vi "majchambre.vi"() -> ()   [LabVIEW 2015]
uses:
  <vilib>/httpClient/LabVIEWHTTPClient.lvlib
panel:
  in  "OK Button 4":bool
  in  "OK Button 3":bool
  in  "String 2":string
  in  "String":string
  in  "Combo Box":string(combo)
  in  "OK Button 2":bool
  in  "OK Button":bool
  # "Choisir  chambre"
  # "Nom chambre"
  # "Description chambre"
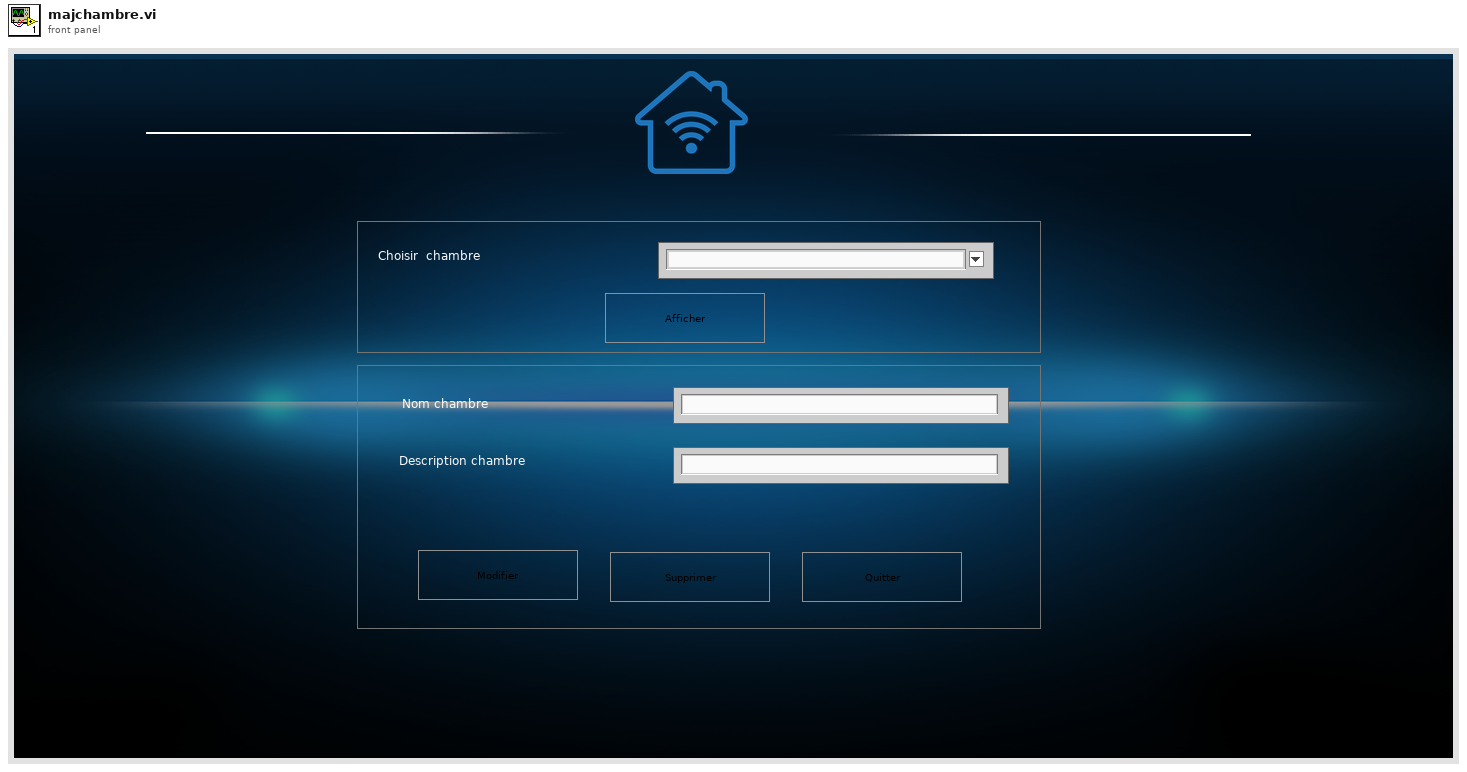
[diagram p1: front panel]
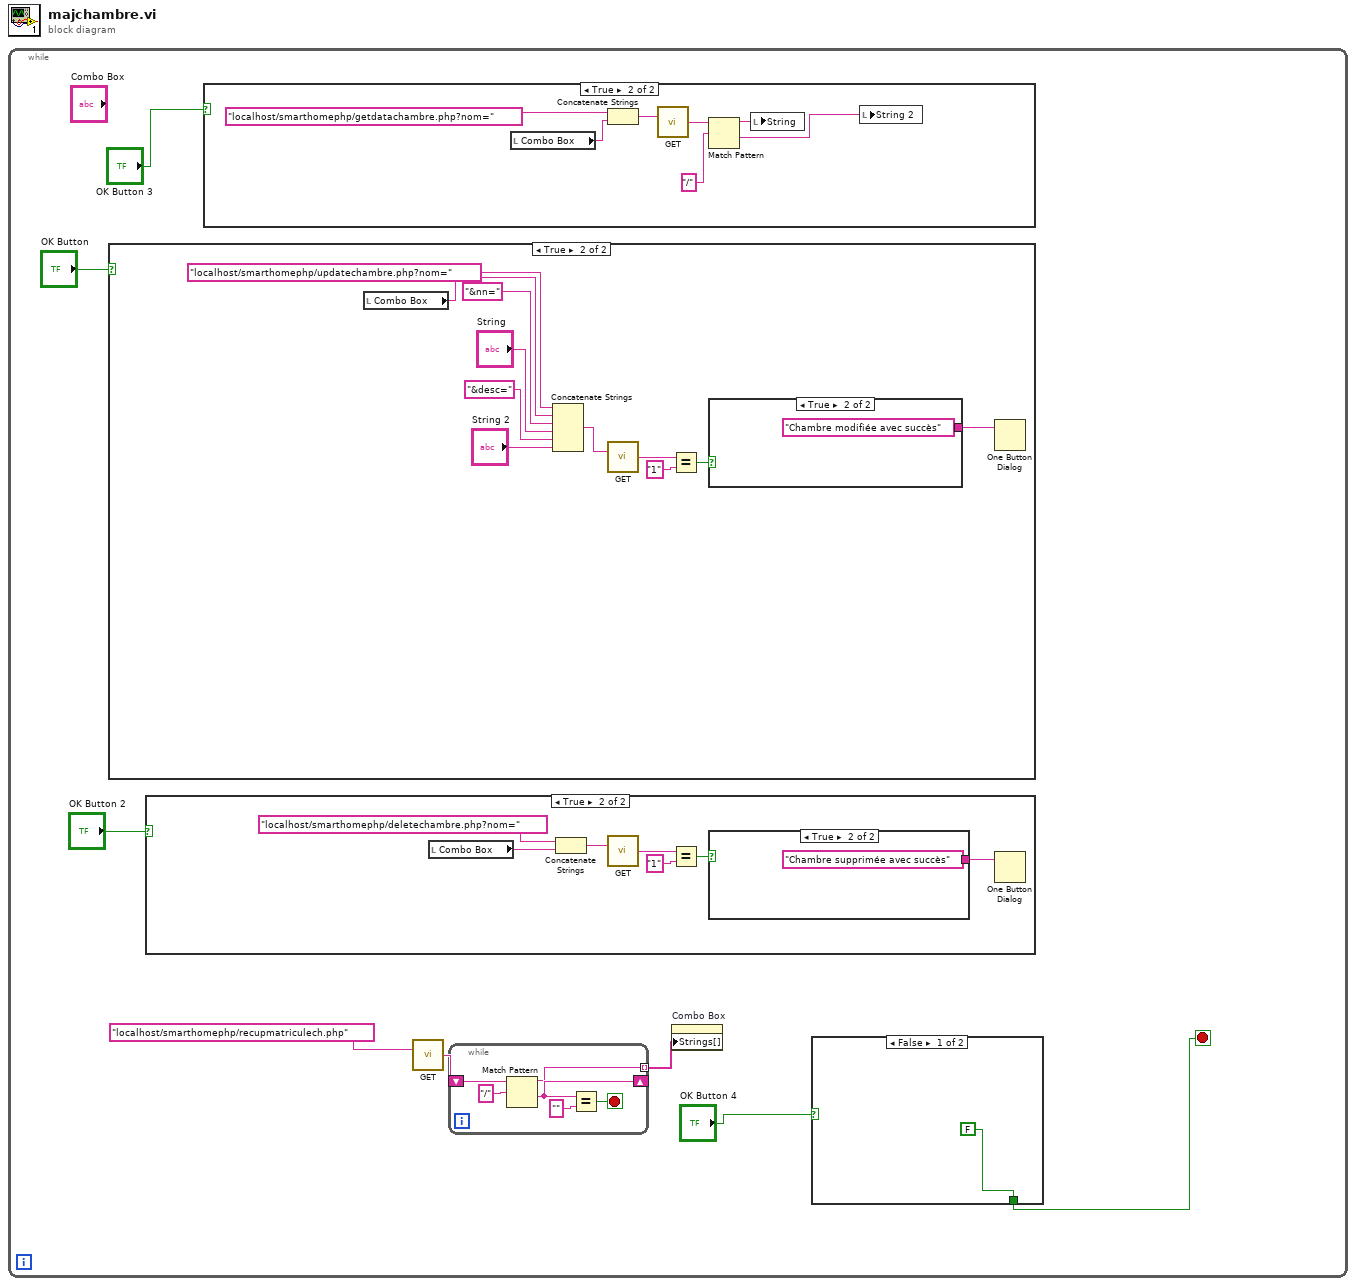
[diagram p0: block diagram]
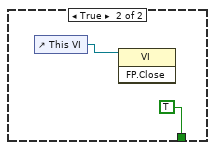
[diagram p2: hidden frame]
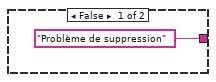
[diagram p4: hidden frame]
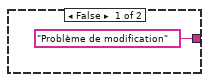
[diagram p6: hidden frame]
diagram:
  n1 = while {
    stop <- w1 stop-if-true
    n2 = case shown="True" "OK Button" {
      frame False {
      }
      frame True {
        n3 = local read "Combo Box"() -> (w36:string)
        n4 = Concatenate Strings("localhost/smarthomephp/updatechambre.php?nom=", w36, "&nn=", "String", "&desc=", "String 2") -> (w31:string)
        n5 = call <vilib>:"GET.vi"("url"=w31) -> ("body"=w30:string)  [unwired: 11 in, 3 out]
        n6 = Equal?(x=w30, y="1") -> (x = y?=w28:bool)
        n7 = case shown="True" w28 {
          tunnel: ["Problème de modification" "Chambre modifiée avec succès"] -> w27
          frame False {
          }
          frame True {
          }
        }
        n8 = One Button Dialog(message=w27) -> ()  [unwired: 1 in, 1 out]
      }
    }
    n9 = case shown="True" "OK Button 2" {
      frame False {
      }
      frame True {
        n10 = local read "Combo Box"() -> (w19:string)
        n11 = Concatenate Strings("localhost/smarthomephp/deletechambre.php?nom=", w19) -> (w18:string)
        n12 = call <vilib>:"GET.vi"("url"=w18) -> ("body"=w21:string)  [unwired: 11 in, 3 out]
        n13 = Equal?(x=w21, y="1") -> (x = y?=w23:bool)
        n14 = case shown="True" w23 {
          tunnel: ["Problème de suppression" "Chambre supprimée avec succès"] -> w24
          frame False {
          }
          frame True {
          }
        }
        n15 = One Button Dialog(message=w24) -> ()  [unwired: 1 in, 1 out]
      }
    }
    n16 = case shown="True" "OK Button 3" {
      frame False {
      }
      frame True {
        n17 = local read "Combo Box"() -> (w45:string)
        n18 = Concatenate Strings("localhost/smarthomephp/getdatachambre.php?nom=", w45) -> (w44:string)
        n19 = call <vilib>:"GET.vi"("url"=w44) -> ("body"=w43:string)  [unwired: 11 in, 3 out]
        n20 = Match Pattern(string=w43, regular expression="/") -> (before substring=w42:string, after substring=w40:string)  [unwired: 1 in, 2 out]
        n21 = local write "String"(w42) -> ()
        n22 = local write "String 2"(w40) -> ()
      }
    }
    n23 = call <vilib>:"GET.vi"("url"="localhost/smarthomephp/recupmatriculech.php") -> ("body"=w4:string)  [unwired: 11 in, 3 out]
    n24 = while {
      shift-right: [w14] -> _
      shift-left: w4 -> [w16]
      tunnel: [w12] -> w5 mode=indexing
      stop <- w13 stop-if-true
      n25 = Match Pattern(string=w16, regular expression="/") -> (before substring=w12:string, after substring=w14:string)  [unwired: 1 in, 2 out]
      n26 = Equal?(x=w14, y="") -> (x = y?=w13:bool)
    }
    n27 = property on="Combo Box" class="CmbBox"("Strings[]"=w5) -> ()  [unwired: 2 in, 2 out]
    n28 = case shown="False" "OK Button 4" {
      tunnel: [FALSE TRUE] -> w1
      frame False {
      }
      frame True {
        n29 = control-ref of="This VI"() -> (w11:refnum<vi>)
        n30 = invoke class="VI" method="FP.Close"(reference=w11) -> ()  [unwired: 2 in, 3 out]
      }
    }
  }
